vi "log analysis_gps.vi"() -> ()   [LabVIEW 2018] (continued)
0.0959,0.0768,0.1404,0.1455,4.9710,0f000001,0*c3454afa\n\tsystem status\tnormal 2 28.000000 0 0\trobot status\t312.499994\t49.181058\t10.952900\t-0.801069\t1.536454\t-28.115818\t0.278000\t0.033000\n\t\n15:25:42.1\tlog_raw\tgps_raw\t#INSPVAXA,USB3,0,48.5,FINESTEERING,2107,282360.150,02000000,471d,15824;INS_ALIGNMENT_COMPLETE,INS_RTKFIXED,37.37057265059,126.72436438219,10.9582,22.3000,-0.1754,0.2257,0.0186,-0.842848206,1.417409471,118.070069819,0.4412,0.2945,0.5472,0.1174,0.0950,0.0769,0.1402,0.1453,4.9710,0f000001,0*6a16ee00\n\tsystem status\tnormal 2 28.000000 0 0\trobot status\t312.617584\t49.099743\t10.958200\t-0.842848\t1.417409\t-28.070070\t0.252000\t0.062000\n\t\n15:25:42.6\tlog_raw\tgps_raw\t#INSPVAXA,USB3,0,48.5,FINESTEERING,2107,282360.650,02000000,471d,15824;INS_ALIGNMENT_COMPLETE,INS_RTKFIXED,37.37057191747,126.72436570845,10.9626,22.3000,-0.1784,0.2288,0.0199,-0.831650114,1.387719615,118.066694933,0.4412,0.2945,0.5472,0.1174,0.0950,0.0769,0.1402,0.1453,4.9710,0f000001,0*684747fc\n\tsystem status\tnormal 2 28.000000 0 0\trobot status\t312.735062\t49.018374\t10.962600\t-0.831650\t1.387720\t-28.066695\t0.284000\t0.026000\n\t\n15:25:43.1\tlog_raw\tgps_raw\t\tsystem status\tnormal 2 28.000000 0 0\trobot status\t312.853231\t48.935714\t10.967100\t-0.777129\t1.230060\t-28.133928\t0.295000\t-0.003000\n\t\n15:25:43.6\tlog_raw\tgps_raw\t#INSPVAXA,USB3,0,48.0,FINESTEERING,2107,282361.650,02000000,471d,15824;INS_ALIGNMENT_COMPLETE,INS_RTKFIXED,37.37057042530,126.72436839921,10.9712,22.3000,-0.1758,0.2244,0.0130,-0.782174586,1.064389692,118.205019127,0.4403,0.2942,0.5440,0.1166,0.0940,0.0770,0.1401,0.1452,4.9712,0f000001,0*a289776d\n\tsystem status\tnormal 2 28.000000 0 0\trobot status\t312.973405\t48.852757\t10.971200\t-0.782175\t1.064390\t-28.205019\t0.294000\t0.001000\n\t\n15:25:44.1\tlog_raw\tgps_raw\t#INSPVAXA,USB3,0,52.0,FINESTEERING,2107,282362.150,02000000,471d,15824;INS_ALIGNMENT_COMPLETE,INS_RTKFIXED,37.37056968661,126.72436971158,10.9754,22.3000,-0.1789,0.2227,0.0149,-0.712007512,1.145542222,118.217293959,0.4394,0.2937,0.5418,0.1158,0.0932,0.0771,0.1400,0.1450,4.9721,0f000001,0*3affd318\n\tsystem status\tnormal 2 28.000000 0 0\trobot status\t313.089653\t48.770770\t10.975400\t-0.712008\t1.145542\t-28.217294\t0.297000\t-0.006000\n\t\n15:25:44.6\tlog_raw\tgps_raw\t#INSPVAXA,USB3,0,52.0,FINESTEERING,2107,282362.650,02000000,471d,15824;INS_ALIGNMENT_COMPLETE,INS_RTKFIXED,37.37056893906,126.72437106065,10.9790,22.3000,-0.1744,0.2169,0.0071,-0.647011256,1.079419362,118.301292650,0.4394,0.2937,0.5418,0.1158,0.0932,0.0771,0.1400,0.1450,4.9721,0f000001,0*1e26d504\n\tsystem status\tnormal 2 28.000000 0 0\trobot status\t313.209151\t48.687799\t10.979000\t-0.647011\t1.079419\t-28.301293\t0.295000\t-0.013000\n\t\n15:25:45.1\tlog_raw\tgps_raw\t#INSPVAXA,USB3,0,52.5,FINESTEERING,2107,282363.150,02000000,471d,15824;INS_ALIGNMENT_COMPLETE,INS_RTKFIXED,37.37056818219,126.72437236922,10.9848,22.3000,-0.1880,0.2251,0.0164,-0.692024407,1.031121061,118.296623598,0.4394,0.2937,0.5418,0.1158,0.0932,0.0771,0.1400,0.1450,4.9721,0f000001,0*fbc0c197\n\tsystem status\tnormal 2 28.000000 0 0\trobot status\t313.325062\t48.603793\t10.984800\t-0.692024\t1.031121\t-28.296624\t0.300000\t0.002000\n\t\n15:25:45.6\tlog_raw\tgps_raw\t#INSPVAXA,USB3,0,52.5,FINESTEERING,2107,282363.650,02000000,471d,15824;INS_ALIGNMENT_COMPLETE,INS_RTKFIXED,37.37056736764,126.72437362581,10.9943,22.3000,-0.1838,0.2175,0.0187,-0.622586307,1.194821727,118.320117324,0.4394,0.2937,0.5418,0.1158,0.0932,0.0771,0.1400,0.1450,4.9721,0f000001,0*9ae06ad3\n\tsystem status\tnormal 2 28.000000 0 0\trobot status\t313.436369\t48.513387\t10.994300\t-0.622586\t1.194822\t-28.320117\t0.300000\t-0.003000\n\t\n15:25:46.1\tlog_raw\tgps_raw\t#INSPVAXA,USB3,0,46.5,FINESTEERING,2107,282364.150,02000000,471d,15824;INS_ALIGNMENT_COMPLETE,INS_RTKFIXED,37.37056657190,126.72437491440,11.0023,22.3000,-0.1853,0.2142,0.0193,-0.566287022,1.525613258,118.367713694,0.4907,0.3307,0.5859,0.1218,0.0978,0.0797,0.1410,0.1460,4.9751,0f000001,0*d0324f7d\n\tsystem status\tnormal 2 28.000000 0 0\trobot status\t313.550510\t48.425068\t11.002300\t-0.566287\t1.525613\t-28.367714\t0.297000\t-0.005000\n\t\n15:25:46.6\tlog_raw\tgps_raw\t#INSPVAXA,USB3,0,46.5,FINESTEERING,2107,282364.650,02000000,471d,15824;INS_ALIGNMENT_COMPLETE,INS_RTKFIXED,37.37056585214,126.72437630982,11.0047,22.3000,-0.1882,0.2248,0.0125,-0.569851294,1.528591804,118.479722218,0.4907,0.3307,0.5859,0.1218,0.0978,0.0797,0.1410,0.1460,4.9751,0f000001,0*9a426144\n\tsystem status\tnormal 2 28.000000 0 0\trobot status\t313.674114\t48.345181\t11.004700\t-0.569851\t1.528592\t-28.479722\t0.298000\t-0.001000\n\t\n15:25:47.1\tlog_raw\tgps_raw\t\tsystem status\tnormal 2 28.100000 0 0\trobot status\t313.794701\t48.266052\t11.006300\t-0.641358\t1.532620\t-28.563005\t0.302000\t-0.002000\n\t\n15:25:47.6\tlog_raw\tgps_raw\t#INSPVAXA,USB3,0,48.5,FINESTEERING,2107,282365.650,02000000,471d,15824;INS_ALIGNMENT_COMPLETE,INS_RTKFIXED,37.37056440793,126.72437904086,11.0071,22.3000,-0.1949,0.2319,0.0130,-0.541846536,1.457071221,118.616213426,0.4699,0.3127,0.5753,0.1175,0.0943,0.0785,0.1406,0.1454,4.9762,0f000001,0*40288813\n\tsystem status\tnormal 2 28.000000 0 0\trobot status\t313.916025\t48.184886\t11.007100\t-0.541847\t1.457071\t-28.616213\t0.302000\t-0.003000\n\t\n15:25:48.1\tlog_raw\tgps_raw\t\tsystem status\tnormal 2 28.000000 0 0\trobot status\t314.039024\t48.101275\t11.008300\t-0.456498\t1.022290\t-28.706558\t0.301000\t-0.003000\n\t\n15:25:48.6\tlog_raw\tgps_raw\t#INSPVAXA,USB3,0,51.0,FINESTEERING,2107,282366.650,02000000,471d,15824;INS_ALIGNMENT_COMPLETE,INS_RTKFIXED,37.37056291329,126.72438179261,11.0096,22.3000,-0.1917,0.2323,0.0080,-0.472728145,0.808367431,118.811459279,0.4569,0.3025,0.5669,0.1155,0.0932,0.0778,0.1406,0.1452,4.9769,0f000001,0*4a7ebce1\n\tsystem status\tnormal 2 28.000000 0 0\trobot status\t314.159770\t48.018995\t11.009600\t-0.472728\t0.808367\t-28.811459\t0.299000\t-0.008000\n\t\n15:25:49.1\tlog_raw\tgps_raw\t#INSPVAXA,USB3,0,52.5,FINESTEERING,2107,282367.150,02000000,471d,15824;INS_ALIGNMENT_COMPLETE,INS_RTKFIXED,37.37056215950,126.72438315251,11.0104,22.3000,-0.1905,0.2375,-0.0008,-0.383174802,0.623906770,118.905218595,0.4483,0.2967,0.5601,0.1147,0.0932,0.0773,0.1406,0.1452,4.9782,0f000001,0*ea495475\n\tsystem status\tnormal 2 28.000000 0 0\trobot status\t314.280228\t47.935332\t11.010400\t-0.383175\t0.623907\t-28.905219\t0.300000\t0.000000\n\t\n15:25:49.6\tlog_raw\tgps_raw\t#INSPVAXA,USB3,0,52.5,FINESTEERING,2107,282367.650,02000000,471d,15824;INS_ALIGNMENT_COMPLETE,INS_RTKFIXED,37.37056140665,126.72438451966,11.0108,22.3000,-0.1856,0.2294,0.0072,-0.390392792,0.506918836,119.017967456,0.4483,0.2967,0.5601,0.1147,0.0932,0.0773,0.1406,0.1452,4.9782,0f000001,0*a0cb1e22\n\tsystem status\tnormal 2 28.000000 0 0\trobot status\t314.401328\t47.851772\t11.010800\t-0.390393\t0.506919\t-29.017967\t0.295000\t-0.009000\n\t\n15:25:50.1\tlog_raw\tgps_raw\t#INSPVAXA,USB3,0,51.0,FINESTEERING,2107,282368.150,02000000,471d,15824;INS_ALIGNMENT_COMPLETE,INS_RTKFIXED,37.37056062590,126.72438588956,11.0109,22.3000,-0.1908,0.2384,0.0056,-0.245023334,0.482634279,119.176381690,0.4426,0.2937,0.5546,0.1146,0.0935,0.0770,0.1406,0.1452,4.9797,0f000001,0*61c8f471\n\tsystem status\tnormal 2 28.100000 0 0\trobot status\t314.522672\t47.765117\t11.010900\t-0.245023\t0.482634\t-29.176382\t0.301000\t-0.006000\n\t\n15:25:50.6\tlog_raw\tgps_raw\t\tsystem status\tnormal 2 28.000000 0 0\trobot status\t314.639459\t47.680741\t11.011100\t-0.155698\t0.523708\t-29.322196\t0.294000\t-0.012000\n\t\n15:25:51.1\tlog_raw\tgps_raw\t\tsystem status\tnormal 2 28.100000 0 0\trobot status\t314.757852\t47.595867\t11.011700\t-0.203616\t0.629165\t-29.462789\t0.298000\t-0.005000\n\t\n15:25:51.6\tlog_raw\tgps_raw\t\tsystem status\tnormal 2 28.000000 0 0\trobot status\t314.875057\t47.511316\t11.012200\t-0.096345\t0.825852\t-29.603097\t0.305000\t-0.002000\n\t\n15:25:52.1\tlog_raw\tgps_raw\t#INSPVAXA,USB3,0,49.0,FINESTEERING,2107,282370.150,02000000,471d,15824;INS_ALIGNMENT_COMPLETE,INS_RTKFIXED,37.37055758372,126.72439118773,11.0127,22.3000,-0.1993,0.2333,0.0205,-0.126523860,1.017645385,119.745065881,0.4369,0.2920,0.5469,0.1146,0.0935,0.0767,0.1404,0.1452,4.9818,0f000001,0*3c99dcc1\n\tsystem status\tnormal 2 28.100000 0 0\trobot status\t314.991975\t47.427464\t11.012700\t-0.126524\t1.017645\t-29.745066\t0.303000\t-0.007000\n\t\n15:25:52.6\tlog_raw\tgps_raw\t#INSPVAXA,USB3,0,49.0,FINESTEERING,2107,282370.650,02000000,471d,15824;INS_ALIGNMENT_COMPLETE,INS_RTKFIXED,37.37055683678,126.72439251585,11.0116,22.3000,-0.1882,0.2280,0.0157,-0.028794832,1.243937117,119.855600640,0.4369,0.2920,0.5469,0.1146,0.0935,0.0767,0.1404,0.1452,4.9818,0f000001,0*7496fdf6\n\tsystem status\tnormal 2 28.000000 0 0\trobot status\t315.109617\t47.344561\t11.011600\t-0.028795\t1.243937\t-29.855601\t0.298000\t-0.003000\n\t\n15:25:53.1\tlog_raw\tgps_raw\t#INSPVAXA,USB3,0,50.0,FINESTEERING,2107,282371.150,02000000,471d,15824;INS_ALIGNMENT_COMPLETE,INS_RTKFIXED,37.37055608815,126.72439385420,11.0119,22.3000,-0.1947,0.2327,0.0119,-0.172585460,1.434683423,119.971021632,0.4362,0.2920,0.5445,0.1145,0.0933,0.0767,0.1403,0.1451,4.9828,0f000001,0*21210484\n\tsystem status\tnormal 2 28.000000 0 0\trobot status\t315.228166\t47.261470\t11.011900\t-0.172585\t1.434683\t-29.971022\t0.298000\t-0.006000\n\t\n15:25:53.6\tlog_raw\tgps_raw\t\tsystem status\tnormal 2 28.000000 0 0\trobot status\t315.345773\t47.177357\t11.014400\t-0.196990\t1.571426\t-30.064709\t0.300000\t-0.003000\n\t\n15:25:54.1\tlog_raw\tgps_raw\t#INSPVAXA,USB3,0,51.5,FINESTEERING,2107,282372.150,02000000,471d,15824;INS_ALIGNMENT_COMPLETE,INS_RTKFIXED,37.37055456936,126.72439651011,11.0164,22.3000,-0.1955,0.2409,0.0111,-0.219662540,1.523066088,120.209141844,0.4362,0.2922,0.5426,0.1144,0.0930,0.0767,0.1402,0.1451,4.9843,0f000001,0*f3fda870\n\tsystem status\tnormal 2 28.000000 0 0\trobot status\t315.463422\t47.092898\t11.016400\t-0.219663\t1.523066\t-30.209142\t0.300000\t-0.003000\n\t\n15:25:54.6\tlog_raw\tgps_raw\t#INSPVAXA,USB3,0,51.5,FINESTEERING,2107,282372.650,02000000,471d,15824;INS_ALIGNMENT_COMPLETE,INS_RTKFIXED,37.37055382453,126.72439783430,11.0178,22.3000,-0.1964,0.2384,0.0010,-0.282113578,1.525554977,120.284642738,0.4362,0.2922,0.5426,0.1144,0.0930,0.0767,0.1402,0.1451,4.9843,0f000001,0*1248182f\n\tsystem status\tnormal 2 28.000000 0 0\trobot status\t315.580717\t47.010229\t11.017800\t-0.282114\t1.525555\t-30.284643\t0.304000\t-0.003000\n\t\n15:25:55.1\tlog_raw\tgps_raw\t\tsystem status\tnormal 2 28.000000 0 0\trobot status\t315.696671\t46.927649\t11.019900\t-0.369047\t1.556384\t-30.408820\t0.302000\t-0.002000\n\t\n15:25:55.6\tlog_raw\tgps_raw\t\tsystem status\tnormal 2 28.000000 0 0\trobot status\t315.812317\t46.846568\t11.022200\t-0.486619\t1.626980\t-30.509329\t0.299000\t-0.001000\n\t\n15:25:56.1\tlog_raw\tgps_raw\t#INSPVAXA,USB3,0,48.5,FINESTEERING,2107,282374.150,02000000,471d,15824;INS_ALIGNMENT_COMPLETE,INS_RTKFIXED,37.37055158865,126.72440177016,11.0240,22.3000,-0.1992,0.2398,-0.0010,-0.425522010,1.592578563,120.559312340,0.4364,0.2923,0.5406,0.1141,0.0924,0.0768,0.1401,0.1450,4.9874,0f000001,0*101c3bdb\n\tsystem status\tnormal 2 28.000000 0 0\trobot status\t315.929349\t46.762068\t11.024000\t-0.425522\t1.592579\t-30.559312\t0.299000\t0.000000\n\t\n15:25:56.6\tlog_raw\tgps_raw\t\tsystem status\tnormal 2 28.000000 0 0\trobot status\t316.042991\t46.678607\t11.025500\t-0.387054\t1.725149\t-30.587652\t0.302000\t0.005000\n\t\n15:25:57.1\tlog_raw\tgps_raw\t#INSPVAXA,USB3,0,51.0,FINESTEERING,2107,282375.150,02000000,471d,15824;INS_ALIGNMENT_COMPLETE,INS_RTKFIXED,37.37055007830,126.72440434973,11.0274,22.3000,-0.1945,0.2378,0.0125,-0.376290277,1.647280363,120.637326967,0.4364,0.2922,0.5400,0.1139,0.0922,0.0768,0.1401,0.1450,4.9889,0f000001,0*67dcfdd6\n\tsystem status\tnormal 2 28.000000 0 0\trobot status\t316.157843\t46.594434\t11.027400\t-0.376290\t1.647280\t-30.637327\t0.300000\t0.005000\n\t\n15:25:57.6\tlog_raw\tgps_raw\t\tsystem status\tnormal 2 28.000000 0 0\trobot status\t316.274584\t46.510665\t11.030000\t-0.408630\t1.445980\t-30.686561\t0.300000\t0.000000\n\t\n15:25:58.1\tlog_raw\tgps_raw\t#INSPVAXA,USB3,0,50.5,FINESTEERING,2107,282376.150,02000000,471d,15824;INS_ALIGNMENT_COMPLETE,INS_RTKFIXED,37.37054852803,126.72440700509,11.0323,22.3000,-0.1988,0.2410,0.0047,-0.545420611,1.322594282,120.751487308,0.4364,0.2922,0.5400,0.1139,0.0922,0.0768,0.1401,0.1450,4.9889,0f000001,0*a32cf91e\n\tsystem status\tnormal 2 28.100000 0 0\trobot status\t316.393051\t46.422369\t11.032300\t-0.545421\t1.322594\t-30.751487\t0.300000\t-0.002000\n\t\n15:25:58.6\tlog_raw\tgps_raw\t\tsystem status\tnormal 2 28.100000 0 0\trobot status\t316.511188\t46.324929\t11.035600\t-0.547076\t1.168807\t-30.825969\t0.296000\t-0.001000\n\t\n15:25:59.1\tlog_raw\tgps_raw\t#INSPVAXA,USB3,0,56.0,FINESTEERING,2107,282377.150,02000000,471d,15824;INS_ALIGNMENT_COMPLETE,INS_RTKFIXED,37.37054676587,126.72440967582,11.0390,22.3000,-0.1999,0.2394,0.0134,-0.643659159,1.057296684,120.890681987,0.4364,0.2922,0.5400,0.1139,0.0922,0.0768,0.1401,0.1450,4.9889,0f000001,0*19d68dee\n\tsystem status\tnormal 2 28.000000 0 0\trobot status\t316.629619\t46.226787\t11.039000\t-0.643659\t1.057297\t-30.890682\t0.302000\t-0.001000\n\t\n15:25:59.6\tlog_raw\tgps_raw\t\tsystem status\tnormal 2 28.000000 0 0\trobot status\t316.748960\t46.127007\t11.042800\t-0.703333\t0.970865\t-30.940874\t0.301000\t-0.001000\n\t\n15:26:00.1\tlog_raw\tgps_raw\t\tsystem status\tnormal 2 28.000000 0 0\trobot status\t316.865490\t46.034320\t11.046500\t-0.687765\t1.023030\t-30.956072\t0.298000\t0.006000\n\t\n15:26:00.6\tlog_raw\tgps_raw\t\tsystem status\tnormal 2 28.000000 0 0\trobot status\t316.977105\t45.965920\t11.049700\t-0.782262\t1.108092\t-31.008444\t0.298000\t0.007000\n\t\n15:26:01.1\tlog_raw\tgps_raw\t\tsystem status\tnormal 2 28.000000 0 0\trobot status\t317.090034\t45.892807\t11.051400\t-0.771591\t1.089832\t-31.020335\t0.298000\t0.004000\n\t\n15:26:01.6\tlog_raw\tgps_raw\t\tsystem status\tnormal 2 28.000000 0 0\trobot status\t317.206952\t45.812611\t11.052200\t-0.744284\t1.080656\t-31.021960\t0.298000\t0.005000\n\t\n15:26:02.1\tlog_raw\tgps_raw\t#INSPVAXA,USB3,0,51.5,FINESTEERING,2107,282380.150,02000000,471d,15824;INS_ALIGNMENT_COMPLETE,INS_RTKFIXED,37.37054231634,126.72441746453,11.0545,22.3000,-0.1950,0.2290,0.0101,-0.779433924,1.099591646,120.976695611,0.4675,0.3093,0.5930,0.1184,0.0970,0.0772,0.1414,0.1460,4.9947,0f000001,0*af9d06d5\n\tsystem status\tnormal 2 28.000000 0 0\trobot status\t317.319531\t45.732932\t11.054500\t-0.779434\t1.099592\t-30.976696\t0.347000\t-0.076000\n\t\n15:26:02.6\tlog_raw\tgps_raw\t\tsystem status\tnormal 2 28.000000 0 0\trobot status\t317.432586\t45.649792\t11.057900\t-0.839077\t1.246140\t-30.921525\t0.333000\t-0.061000\n\t\n15:26:03.1\tlog_raw\tgps_raw\t\tsystem status\tnormal 2 28.000000 0 0\trobot status\t317.550663\t45.559859\t11.060900\t-0.816495\t1.347080\t-30.908043\t0.247000\t0.059000\n\t\n15:26:03.6\tlog_raw\tgps_raw\t\tsystem status\tnormal 2 28.000000 0 0\trobot status\t317.667916\t45.463494\t11.064400\t-0.887391\t1.440630\t-30.847180\t0.259000\t0.059000\n\t\n15:26:04.1\tlog_raw\tgps_raw\t\tsystem status\tnormal 2 28.000000 0 0\trobot status\t317.784177\t45.372249\t11.068000\t-0.895954\t1.399755\t-30.787069\t0.348000\t-0.082000\n\t\n15:26:04.6\tlog_raw\tgps_raw\t\tsystem status\tnormal 2 28.000000 0 0\trobot status\t317.897989\t45.297471\t11.072100\t-0.868246\t1.325384\t-30.710013\t0.268000\t0.039000\n\t\n15:26:05.1\tlog_raw\tgps_raw\t\tsystem status\tnormal 2 28.000000 0 0\trobot status\t318.012551\t45.219365\t11.077100\t-0.737707\t1.224592\t-30.609820\t0.274000\t0.027000\n\t\n15:26:05.6\tlog_raw\tgps_raw\t\tsystem status\tnormal 2 28.000000 0 0\trobot status\t318.126528\t45.138525\t11.083300\t-0.713978\t1.140149\t-30.534342\t0.347000\t-0.089000\n\t\n15:26:06.1\tlog_raw\tgps_raw\t\tsystem status\tnormal 2 28.000000 0 0\trobot status\t318.241724\t45.053708\t11.088800\t-0.781618\t1.201474\t-30.564329\t0.257000\t0.043000\n\t\n15:26:06.6\tlog_raw\tgps_raw\t\tsystem status\tnormal 2 28.000000 0 0\trobot status\t318.360025\t44.958001\t11.094400\t-0.854089\t1.233668\t-30.586480\t0.294000\t-0.009000\n\t\n15:26:07.1\tlog_raw\tgps_raw\t\tsystem status\tnormal 2 28.000000 0 0\trobot status\t318.473921\t44.868063\t11.099900\t-0.830682\t1.383003\t-30.588756\t0.296000\t-0.005000\n\t\n15:26:07.6\tlog_raw\tgps_raw\t\tsystem status\tnormal 2 28.000000 0 0\trobot status\t318.583583\t44.793348\t11.105400\t-0.688458\t1.421619\t-30.626819\t0.293000\t-0.015000\n\t\n15:26:08.1\tlog_raw\tgps_raw\t\tsystem status\tnormal 2 28.100000 0 0\trobot status\t318.695376\t44.715083\t11.110500\t-0.621575\t1.442793\t-30.687734\t0.298000\t-0.012000\n\t\n15:26:08.6\tlog_raw\tgps_raw\t\tsystem status\tnormal 2 28.000000 0 0\trobot status\t318.807113\t44.634368\t11.117200\t-0.699288\t1.578888\t-30.729025\t0.291000\t-0.015000\n\t\n15:26:09.1\tlog_raw\tgps_raw\t\tsystem status\tnormal 2 28.000000 0 0\trobot status\t318.919028\t44.547774\t11.125000\t-0.655876\t1.582589\t-30.761990\t0.296000\t-0.011000\n\t\n15:26:09.6\tlog_raw\tgps_raw\t\tsystem status\tnormal 2 28.000000 0 0\trobot status\t319.034952\t44.448217\t11.133200\t-0.642971\t1.523191\t-30.813225\t0.297000\t-0.014000\n\t\n15:26:10.1\tlog_raw\tgps_raw\t\tsystem status\tnormal 2 28.100000 0 0\trobot status\t319.150075\t44.353379\t11.141000\t-0.602027\t1.630659\t-30.864026\t0.299000\t-0.010000\n\t\n15:26:10.6\tlog_raw\tgps_raw\t\tsystem status\tnormal 2 28.000000 0 0\trobot status\t319.261183\t44.276146\t11.147400\t-0.528294\t1.572516\t-30.922958\t0.298000\t0.000000\n\t\n15:26:11.1\tlog_raw\tgps_raw\t\tsystem status\tnormal 2 28.000000 0 0\trobot status\t319.374097\t44.194709\t11.154200\t-0.383438\t1.395307\t-31.049945\t0.299000\t0.000000\n\t\n15:26:11.7\tlog_raw\tgps_raw\t\tsystem status\tnormal 2 28.000000 0 0\trobot status\t319.488062\t44.108823\t11.159600\t-0.206184\t1.242922\t-31.135620\t0.292000\t-0.007000\n\t\n15:26:12.1\tlog_raw\tgps_raw\t\tsystem status\tnormal 2 28.000000 0 0\trobot status\t319.601847\t44.022896\t11.165400\t-0.173678\t1.198516\t-31.218283\t0.294000\t-0.003000\n\t\n15:26:12.7\tlog_raw\tgps_raw\t\tsystem status\tnormal 2 28.000000 0 0\trobot status\t319.716831\t43.937029\t11.170500\t-0.251651\t1.246692\t-31.292043\t0.296000\t-0.005000\n\t\n15:26:13.2\tlog_raw\tgps_raw\t\tsystem status\tnormal 2 28.000000 0 0\trobot status\t319.831302\t43.849544\t11.176100\t-0.193272\t1.314153\t-31.350185\t0.297000\t-0.010000\n\t\n15:26:13.7\tlog_raw\tgps_raw\t\tsystem status\tnormal 2 28.100000 0 0\trobot status\t319.948465\t43.760462\t11.184100\t-0.050481\t1.406412\t-31.381709\t0.296000\t-0.006000\n\t\n15:26:14.2\tlog_raw\tgps_raw\t\tsystem status\tnormal 2 28.000000 0 0\trobot status\t320.061943\t43.672961\t11.191600\t-0.042890\t1.719894\t-31.413597\t0.301000\t0.003000\n\t\n15:26:14.7\tlog_raw\tgps_raw\t\tsystem status\tnormal 2 28.000000 0 0\trobot status\t320.175399\t43.584307\t11.196800\t-0.016793\t1.699514\t-31.492516\t0.297000\t0.001000\n\t\n15:26:15.2\tlog_raw\tgps_raw\t\tsystem status\tnormal 2 28.000000 0 0\trobot status\t320.290219\t43.495259\t11.202000\t-0.158228\t1.837171\t-31.577321\t0.304000\t0.002000\n\t\n15:26:15.7\tlog_raw\tgps_raw\t\tsystem status\tnormal 2 28.000000 0 0\trobot status\t320.403890\t43.407183\t11.206700\t-0.121054\t1.987495\t-31.576185\t0.295000\t0.005000\n\t\n15:26:16.2\tlog_raw\tgps_raw\t\tsystem status\tnormal 2 28.000000 0 0\trobot status\t320.518730\t43.318566\t11.212000\t-0.192713\t1.993255\t-31.623743\t0.300000\t0.008000\n\t\n15:26:16.7\tlog_raw\tgps_raw\t\tsystem status\tnormal 2 28.000000 0 0\trobot status\t320.635793\t43.229652\t11.218000\t-0.297416\t1.926594\t-31.642658\t0.300000\t-0.001000\n\t\n15:26:17.2\tlog_raw\tgps_raw\t\tsystem status\tnormal 2 28.000000 0 0\trobot status\t320.751780\t43.139819\t11.224000\t-0.293698\t2.010038\t-31.639513\t0.303000\t0.005000\n\t\n15:26:17.7\tlog_raw\tgps_raw\t\tsystem status\tnormal 2 28.000000 0 0\trobot status\t320.866959\t43.051021\t11.228800\t-0.252225\t1.853648\t-31.644727\t0.312000\t0.000000\n\t\n15:26:18.2\tlog_raw\tgps_raw\t#INSPVAXA,USB3,0,53.0,FINESTEERING,2107,282396.200,02000000,471d,15824;INS_ALIGNMENT_COMPLETE,INS_RTKFIXED,37.37051727534,126.72445893614,11.2346,22.3000,-0.2149,0.2448,0.0105,-0.230381953,1.670919034,121.706042723,0.4454,0.2945,0.5444,0.1167,0.0933,0.0771,0.1396,0.1448,5.0169,0f000001,0*e3a105a8\n\tsystem status\tnormal 2 28.000000 0 0\trobot status\t320.993018\t42.953626\t11.234600\t-0.230382\t1.670919\t-31.706043\t0.300000\t0.002000\n\t\n15:26:18.7\tlog_raw\tgps_raw\t\tsystem status\tnormal 2 28.000000 0 0\trobot status\t321.098911\t42.873834\t11.238800\t-0.374769\t1.739257\t-31.716837\t0.308000\t0.000000\n\t\n15:26:19.2\tlog_raw\tgps_raw\t\tsystem status\tnormal 2 28.000000 0 0\trobot status\t321.215034\t42.784862\t11.243700\t-0.317896\t1.583496\t-31.672183\t0.300000\t0.004000\n\t\n15:26:19.7\tlog_raw\tgps_raw\t\tsystem status\tnormal 2 28.000000 0 0\trobot status\t321.328995\t42.697954\t11.248100\t-0.292274\t1.413082\t-31.609032\t0.276000\t0.045000\n\t\n15:26:20.2\tlog_raw\tgps_raw\t\tsystem status\tnormal 2 28.000000 0 0\trobot status\t321.443612\t42.609385\t11.252400\t-0.217796\t1.413222\t-31.467886\t0.278000\t0.035000\n\t\n15:26:20.7\tlog_raw\tgps_raw\t\tsystem status\tnormal 2 28.000000 0 0\trobot status\t321.559858\t42.520982\t11.255400\t-0.213988\t1.321824\t-31.289097\t0.239000\t0.085000\n\t\n15:26:21.2\tlog_raw\tgps_raw\t\tsystem status\tnormal 2 28.000000 0 0\trobot status\t321.673832\t42.434194\t11.258900\t-0.220342\t1.308636\t-31.041861\t0.293000\t0.016000\n\t\n15:26:21.7\tlog_raw\tgps_raw\t#INSPVAXA,USB3,0,52.5,FINESTEERING,2107,282399.700,02000000,471d,15824;INS_ALIGNMENT_COMPLETE,INS_RTKFIXED,37.37051173912,126.72446803450,11.2629,22.3000,-0.2157,0.2432,0.0104,-0.126649868,1.183808073,120.810959551,0.4494,0.2941,0.5444,0.1155,0.0921,0.0775,0.1396,0.1447,5.0208,0f000001,0*57a15611\n\tsystem status\tnormal 2 28.000000 0 0\trobot status\t321.798936\t42.339160\t11.262900\t-0.126650\t1.183808\t-30.810960\t0.289000\t0.028000\n\t\n15:26:22.2\tlog_raw\tgps_raw\t#INSPVAXA,USB3,0,51.5,FINESTEERING,2107,282400.200,02000000,471d,15824;INS_ALIGNMENT_COMPLETE,INS_RTKFIXED,37.37051098079,126.72446931042,11.2663,22.3000,-0.2068,0.2423,0.0047,-0.194058602,1.122857123,120.589823258,0.4487,0.2937,0.5447,0.1150,0.0920,0.0775,0.1397,0.1447,5.0216,0f000001,0*c9fba93a\n\tsystem status\tnormal 2 28.000000 0 0\trobot status\t321.911955\t42.254993\t11.266300\t-0.194059\t1.122857\t-30.589823\t0.284000\t0.024000\n\t\n15:26:22.7\tlog_raw\tgps_raw\t#INSPVAXA,USB3,0,51.5,FINESTEERING,2107,282400.700,02000000,471d,15824;INS_ALIGNMENT_COMPLETE,INS_RTKFIXED,37.37051023771,126.72447057615,11.2691,22.3000,-0.2018,0.2421,0.0003,-0.178083607,1.252069735,120.254195677,0.4487,0.2937,0.5447,0.1150,0.0920,0.0775,0.1397,0.1447,5.0216,0f000001,0*c019cdcb\n\tsystem status\tnormal 2 28.000000 0 0\trobot status\t322.024071\t42.172518\t11.269100\t-0.178084\t1.252070\t-30.254196\t0.274000\t0.045000\n\t\n15:26:23.2\tlog_raw\tgps_raw\t\tsystem status\tnormal 2 27.900000 0 0\trobot status\t322.123807\t42.099686\t11.272300\t-0.161582\t1.307019\t-29.978398\t0.308000\t-0.002000\n\t\n15:26:23.7\tlog_raw\tgps_raw\t\tsystem status\tnormal 2 28.000000 0 0\trobot status\t322.238275\t42.017640\t11.276500\t-0.061771\t1.314666\t-29.738310\t0.279000\t0.036000\n\t\n15:26:24.2\tlog_raw\tgps_raw\t\tsystem status\tnormal 2 28.000000 0 0\trobot status\t322.352343\t41.937206\t11.280200\t-0.171851\t1.578799\t-29.480802\t0.412000\t-0.174000\n\t\n15:26:24.7\tlog_raw\tgps_raw\t#INSPVAXA,USB3,0,52.0,FINESTEERING,2107,282402.700,02000000,471d,15824;INS_ALIGNMENT_COMPLETE,INS_RTKFIXED,37.37050732665,126.72447567900,11.2840,22.3000,-0.1846,0.2304,0.0147,-0.197464539,1.720744587,119.244672502,0.4474,0.2933,0.5456,0.1143,0.0919,0.0775,0.1398,0.1447,5.0227,0f000001,0*ef6b078e\n\tsystem status\tnormal 2 28.000000 0 0\trobot status\t322.476073\t41.849418\t11.284000\t-0.197465\t1.720745\t-29.244673\t0.290000\t0.025000\n\t\n15:26:25.2\tlog_raw\tgps_raw\t\tsystem status\tnormal 2 28.000000 0 0\trobot status\t322.579374\t41.776811\t11.285800\t-0.232380\t1.437411\t-29.131770\t0.279000\t0.023000\n\t\n15:26:25.7\tlog_raw\tgps_raw\t#INSPVAXA,USB3,0,51.0,FINESTEERING,2107,282403.700,02000000,471d,15824;INS_ALIGNMENT_COMPLETE,INS_RTKFIXED,37.37050587454,126.72447826035,11.2883,22.3000,-0.1895,0.2228,0.0117,-0.041463128,1.413686081,119.013719695,0.4466,0.2931,0.5458,0.1142,0.0920,0.0774,0.1398,0.1448,5.0238,0f000001,0*aa5be0c8\n\tsystem status\tnormal 2 28.000000 0 0\trobot status\t322.704725\t41.688247\t11.288300\t-0.041463\t1.413686\t-29.013720\t0.280000\t0.023000\n\t\n15:26:26.2\tlog_raw\tgps_raw\t\tsystem status\tnormal 2 28.000000 0 0\trobot status\t322.807611\t41.615847\t11.290100\t0.014448\t1.226451\t-28.973744\t0.269000\t0.043000\n\t\n15:26:26.7\tlog_raw\tgps_raw\t\tsystem status\tnormal 2 28.000000 0 0\trobot status\t322.922819\t41.536064\t11.293200\t-0.047041\t1.026542\t-28.942700\t0.261000\t0.062000\n\t\n15:26:27.2\tlog_raw\tgps_raw\t#INSPVAXA,USB3,0,53.0,FINESTEERING,2107,282405.200,02000000,471d,15824;INS_ALIGNMENT_COMPLETE,INS_RTKFIXED,37.37050369833,126.72448216938,11.2960,22.3000,-0.1948,0.2280,0.0025,-0.062260759,1.020577864,118.930310663,0.4445,0.2927,0.5458,0.1142,0.0920,0.0773,0.1398,0.1448,5.0258,0f000001,0*8918fe41\n\tsystem status\tnormal 2 28.000000 0 0\trobot status\t323.050980\t41.446708\t11.296000\t-0.062261\t1.020578\t-28.930311\t0.346000\t-0.071000\n\t\n15:26:27.7\tlog_raw\tgps_raw\t\tsystem status\tnormal 2 28.000000 0 0\trobot status\t323.157063\t41.374190\t11.297300\t8.474600E-5\t0.954576\t-28.962463\t0.297000\t-0.005000\n\t\n15:26:28.2\tlog_raw\tgps_raw\t#INSPVAXA,USB3,0,49.0,FINESTEERING,2107,282406.200,02000000,471d,15824;INS_ALIGNMENT_COMPLETE,INS_RTKFIXED,37.37050223457,126.72448478438,11.2989,22.3000,-0.1940,0.2271,0.0004,0.403911528,1.100287176,119.003406163,0.4431,0.2925,0.5454,0.1141,0.0922,0.0772,0.1398,0.1448,5.0266,0f000001,0*9acaefa2\n\tsystem status\tnormal 2 28.100000 0 0\trobot status\t323.282613\t41.284244\t11.298900\t0.403912\t1.100287\t-29.003406\t0.308000\t-0.008000\n\t\n15:26:28.7\tlog_raw\tgps_raw\t#INSPVAXA,USB3,0,49.0,FINESTEERING,2107,282406.700,02000000,471d,15824;INS_ALIGNMENT_COMPLETE,INS_RTKFIXED,37.37050154645,126.72448605087,11.3007,22.3000,-0.1906,0.2211,-0.0024,0.198399759,1.155504209,119.019429949,0.4431,0.2925,0.5454,0.1141,0.0922,0.0772,0.1398,0.1448,5.0266,0f000001,0*2b05d55f\n\tsystem status\tnormal 2 28.000000 0 0\trobot status\t323.394796\t41.207869\t11.300700\t0.198400\t1.155504\t-29.019430\t0.300000\t-0.005000\n\t\n15:26:29.2\tlog_raw\tgps_raw\t#INSPVAXA,USB3,0,49.5,FINESTEERING,2107,282407.200,02000000,471d,15824;INS_ALIGNMENT_COMPLETE,INS_RTKFIXED,37.37050082511,126.72448737364,11.3024,22.3000,-0.1843,0.2252,0.0031,0.001432132,1.154226626,118.999213590,0.4420,0.2924,0.5450,0.1140,0.0921,0.0771,0.1398,0.1448,5.0273,0f000001,0*acf3bb7b\n\tsystem status\tnormal 2 28.100000 0 0\trobot status\t323.511965\t41.127807\t11.302400\t0.001432\t1.154227\t-28.999214\t0.299000\t-0.008000\n\t\n15:26:29.7\tlog_raw\tgps_raw\t#INSPVAXA,USB3,0,49.5,FINESTEERING,2107,282407.700,02000000,471d,15824;INS_ALIGNMENT_COMPLETE,INS_RTKFIXED,37.37050009749,126.72448866196,11.3047,22.3000,-0.1922,0.2264,0.0013,0.031954534,1.373571777,119.029897417,0.4420,0.2924,0.5450,0.1140,0.0921,0.0771,0.1398,0.1448,5.0273,0f000001,0*4feaee25\n\tsystem status\tnormal 2 28.000000 0 0\trobot status\t323.626082\t41.047048\t11.304700\t0.031955\t1.373572\t-29.029897\t0.304000\t-0.002000\n\t\n15:26:30.2\tlog_raw\tgps_raw\t\tsystem status\tnormal 2 28.000000 0 0\trobot status\t323.727747\t40.974413\t11.307100\t0.072493\t1.528107\t-29.075426\t0.301000\t-0.002000\n\t\n15:26:30.7\tlog_raw\tgps_raw\t#INSPVAXA,USB3,0,49.5,FINESTEERING,2107,282408.700,02000000,471d,15824;INS_ALIGNMENT_COMPLETE,INS_RTKFIXED,37.37049862952,126.72449128459,11.3098,22.3000,-0.1866,0.2253,0.0102,0.047127376,1.614716400,119.167288999,0.4410,0.2922,0.5445,0.1140,0.0921,0.0770,0.1398,0.1448,5.0281,0f000001,0*196c2f22\n\tsystem status\tnormal 2 28.000000 0 0\trobot status\t323.858391\t40.884117\t11.309800\t0.047127\t1.614716\t-29.167289\t0.303000\t-0.012000\n\t\n15:26:31.2\tlog_raw\tgps_raw\t#INSPVAXA,USB3,0,47.5,FINESTEERING,2107,282409.200,02000000,471d,15824;INS_ALIGNMENT_COMPLETE,INS_RTKFIXED,37.37049789341,126.72449262767,11.3125,22.3000,-0.1999,0.2359,0.0079,-0.178457330,1.548416838,119.244672995,0.4408,0.2923,0.5442,0.1140,0.0922,0.0770,0.1398,0.1448,5.0295,0f000001,0*fefe7bbe\n\tsystem status\tnormal 2 28.000000 0 0\trobot status\t323.977358\t40.802415\t11.312500\t-0.178457\t1.548417\t-29.244673\t0.302000\t0.000000\n\t\n15:26:31.7\tlog_raw\tgps_raw\t\tsystem status\tnormal 2 28.100000 0 0\trobot status\t324.083822\t40.729055\t11.315700\t-0.361621\t1.540910\t-29.327056\t0.299000\t-0.004000\n\t\n15:26:32.2\tlog_raw\tgps_raw\t\tsystem status\tnormal 2 28.000000 0 0\trobot status\t324.201244\t40.646211\t11.320200\t-0.395668\t1.402025\t-29.391054\t0.295000\t-0.006000\n\t\n15:26:32.7\tlog_raw\tgps_raw\t#INSPVAXA,USB3,0,49.0,FINESTEERING,2107,282410.700,02000000,471d,15824;INS_ALIGNMENT_COMPLETE,INS_RTKFIXED,37.37049566854,126.72449665280,11.3239,22.3000,-0.1868,0.2363,0.0016,-0.505574846,1.345277164,119.533703259,0.4402,0.2922,0.5436,0.1139,0.0922,0.0769,0.1398,0.1447,5.0311,0f000001,0*6012c6b0\n\tsystem status\tnormal 2 28.000000 0 0\trobot status\t324.333898\t40.555475\t11.323900\t-0.505575\t1.345277\t-29.533703\t0.305000\t-0.006000\n\t\n15:26:33.2\tlog_raw\tgps_raw\t#INSPVAXA,USB3,0,50.0,FINESTEERING,2107,282411.200,02000000,471d,15824;INS_ALIGNMENT_COMPLETE,INS_RTKFIXED,37.37049487353,126.72449799751,11.3279,22.3000,-0.1792,0.2394,0.0156,-0.401695145,1.333527826,119.633898753,0.4402,0.2922,0.5436,0.1139,0.0922,0.0769,0.1398,0.1447,5.0311,0f000001,0*2fc42002\n\tsystem status\tnormal 2 28.000000 0 0\trobot status\t324.453010\t40.467237\t11.327900\t-0.401695\t1.333528\t-29.633899\t0.302000\t-0.006000\n\t\n15:26:33.7\tlog_raw\tgps_raw\t#INSPVAXA,USB3,0,50.0,FINESTEERING,2107,282411.700,02000000,471d,15824;INS_ALIGNMENT_COMPLETE,INS_RTKFIXED,37.37049401462,126.72449935015,11.3332,22.3000,-0.1865,0.2337,0.0135,-0.484899234,1.283665048,119.740703059,0.4402,0.2922,0.5436,0.1139,0.0922,0.0769,0.1398,0.1447,5.0311,0f000001,0*1d33eb73\n\tsystem status\tnormal 2 28.000000 0 0\trobot status\t324.572825\t40.371906\t11.333200\t-0.484899\t1.283665\t-29.740703\t0.299000\t-0.008000\n\t\n15:26:34.2\tlog_raw\tgps_raw\t#INSPVAXA,USB3,0,45.5,FINESTEERING,2107,282412.200,02000000,471d,15824;INS_ALIGNMENT_COMPLETE,INS_RTKFIXED,37.37049319930,126.72450071545,11.3390,22.3000,-0.1883,0.2399,0.0132,-0.511269715,1.109019547,119.856142336,0.4907,0.3298,0.5890,0.1210,0.0979,0.0793,0.1408,0.1457,5.0340,0f000001,0*b0282710\n\tsystem status\tnormal 2 28.000000 0 0\trobot status\t324.693761\t40.281414\t11.339000\t-0.511270\t1.109020\t-29.856142\t0.303000\t-0.008000\n\t\n15:26:34.7\tlog_raw\tgps_raw\t#INSPVAXA,USB3,0,45.5,FINESTEERING,2107,282412.700,02000000,471d,15824;INS_ALIGNMENT_COMPLETE,INS_RTKFIXED,37.37049251112,126.72450203682,11.3445,22.3000,-0.1885,0.2438,0.0204,-0.533735812,1.097181007,119.915108239,0.4907,0.3298,0.5890,0.1210,0.0979,0.0793,0.1408,0.1457,5.0340,0f000001,0*9a141504\n\tsystem status\tnormal 2 28.000000 0 0\trobot status\t324.810806\t40.205032\t11.344500\t-0.533736\t1.097181\t-29.915108\t0.304000\t-0.001000\n\t\n15:26:35.2\tlog_raw\tgps_raw\t#INSPVAXA,USB3,0,46.5,FINESTEERING,2107,282413.200,02000000,471d,15824;INS_ALIGNMENT_COMPLETE,INS_RTKFIXED,37.37049180169,126.72450336418,11.3490,22.3000,-0.1814,0.2477,0.0198,-0.567250496,1.161668497,119.990441604,0.4687,0.3125,0.5782,0.1173,0.0947,0.0780,0.1403,0.1452,5.0347,0f000001,0*907c6878\n\tsystem status\tnormal 2 28.000000 0 0\trobot status\t324.928381\t40.126291\t11.349000\t-0.567250\t1.161668\t-29.990442\t0.304000\t0.007000\n\t\n15:26:35.7\tlog_raw\tgps_raw\t#INSPVAXA,USB3,0,46.5,FINESTEERING,2107,282413.700,02000000,471d,15824;INS_ALIGNMENT_COMPLETE,INS_RTKFIXED,37.37049106798,126.72450467966,11.3532,22.3000,-0.1907,0.2386,0.0196,-0.535844359,1.216959402,120.030591907,0.4687,0.3125,0.5782,0.1173,0.0947,0.0780,0.1403,0.1452,5.0347,0f000001,0*639bb67e\n\tsystem status\tnormal 2 28.000000 0 0\trobot status\t325.044904\t40.044856\t11.353200\t-0.535844\t1.216959\t-30.030592\t0.300000\t0.004000\n\t\n15:26:36.2\tlog_raw\tgps_raw\t#INSPVAXA,USB3,0,51.5,FINESTEERING,2107,282414.200,02000000,471d,15824;INS_ALIGNMENT_COMPLETE,INS_RTKFIXED,37.37049032617,126.72450602273,11.3581,22.3000,-0.1924,0.2499,0.0107,-0.616512696,1.220090147,120.041431319,0.4551,0.3027,0.5696,0.1158,0.0939,0.0773,0.1402,0.1450,5.0349,0f000001,0*41bc56e6\n\tsystem status\tnormal 2 28.000000 0 0\trobot status\t325.163871\t39.962522\t11.358100\t-0.616513\t1.220090\t-30.041431\t0.298000\t0.003000\n\t\n15:26:36.7\tlog_raw\tgps_raw\t#INSPVAXA,USB3,0,51.5,FINESTEERING,2107,282414.700,02000000,471d,15824;INS_ALIGNMENT_COMPLETE,INS_RTKFIXED,37.37048957210,126.72450735141,11.3626,22.3000,-0.1833,0.2491,0.0031,-0.413726161,1.254488863,120.030297293,0.4551,0.3027,0.5696,0.1158,0.0939,0.0773,0.1402,0.1450,5.0349,0f000001,0*52de2f77\n\tsystem status\tnormal 2 28.000000 0 0\trobot status\t325.281563\t39.878827\t11.362600\t-0.413726\t1.254489\t-30.030297\t0.300000\t0.009000\n\t\n15:26:37.2\tlog_raw\tgps_raw\t#INSPVAXA,USB3,0,53.0,FINESTEERING,2107,282415.200,02000000,471d,15824;INS_ALIGNMENT_COMPLETE,INS_RTKFIXED,37.37048882282,126.72450867783,11.3669,22.3000,-0.1974,0.2488,-0.0050,-0.369163180,1.275233001,120.010997524,0.4468,0.2975,0.5625,0.1152,0.0938,0.0768,0.1401,0.1449,5.0346,0f000001,0*63e54e05\n\tsystem status\tnormal 2 28.000000 0 0\trobot status\t325.399055\t39.795664\t11.366900\t-0.369163\t1.275233\t-30.010998\t0.301000\t0.009000\n\t\n15:26:37.7\tlog_raw\tgps_raw\t#INSPVAXA,USB3,0,53.0,FINESTEERING,2107,282415.700,02000000,471d,15824;INS_ALIGNMENT_COMPLETE,INS_RTKFIXED,37.37048807554,126.72451000285,11.3689,22.3000,-0.1889,0.2508,0.0038,-0.308402860,1.363313459,120.035668332,0.4468,0.2975,0.5625,0.1152,0.0938,0.0768,0.1401,0.1449,5.0346,0f000001,0*269cbb1b\n\tsystem status\tnormal 2 28.000000 0 0\trobot status\t325.516423\t39.712723\t11.368900\t-0.308403\t1.363313\t-30.035668\t0.300000\t0.000000\n\t\n15:26:38.2\tlog_raw\tgps_raw\t#INSPVAXA,USB3,0,49.5,FINESTEERING,2107,282416.200,02000000,471d,15824;INS_ALIGNMENT_COMPLETE,INS_RTKFIXED,37.37048732666,126.72451132645,11.3727,22.3000,-0.2024,0.2646,0.0068,-0.344354829,1.559210135,120.006452776,0.4418,0.2949,0.5567,0.1151,0.0940,0.0765,0.1400,0.1448,5.0344,0f000001,0*5f55c88e\n\tsystem status\tnormal 2 28.000000 0 0\trobot status\t325.633666\t39.629604\t11.372700\t-0.344355\t1.559210\t-30.006453\t0.307000\t0.002000\n\t\n15:26:38.7\tlog_raw\tgps_raw\t#INSPVAXA,USB3,0,49.5,FINESTEERING,2107,282416.700,02000000,471d,15824;INS_ALIGNMENT_COMPLETE,INS_RTKFIXED,37.37048655948,126.72451266499,11.3766,22.3000,-0.1941,0.2563,0.0061,-0.377791585,1.578777969,120.002147142,0.4418,0.2949,0.5567,0.1151,0.0940,0.0765,0.1400,0.1448,5.0344,0f000001,0*34897afe\n\tsystem status\tnormal 2 28.000000 0 0\trobot status\t325.752231\t39.544455\t11.376600\t-0.377792\t1.578778\t-30.002147\t0.303000\t0.007000\n\t\n15:26:39.2\tlog_raw\tgps_raw\t\tsystem status\tnormal 2 28.000000 0 0\trobot status\t325.855280\t39.469306\t11.380500\t-0.290945\t1.667739\t-29.924480\t0.258000\t0.066000\n\t\n15:26:39.7\tlog_raw\tgps_raw\t#INSPVAXA,USB3,0,52.5,FINESTEERING,2107,282417.700,02000000,471d,15824;INS_ALIGNMENT_COMPLETE,INS_RTKFIXED,37.37048504382,126.72451529790,11.3842,22.3000,-0.1953,0.2454,0.0181,-0.246271614,1.533033405,119.744385532,0.4392,0.2938,0.5521,0.1151,0.0941,0.0764,0.1399,0.1448,5.0342,0f000001,0*775a7cde\n\tsystem status\tnormal 2 28.000000 0 0\trobot status\t325.985450\t39.376231\t11.384200\t-0.246272\t1.533033\t-29.744386\t0.376000\t-0.093000\n\t\n15:26:40.2\tlog_raw\tgps_raw\t#INSPVAXA,USB3,0,49.5,FINESTEERING,2107,282418.200,02000000,471d,15824;INS_ALIGNMENT_COMPLETE,INS_RTKFIXED,37.37048430161,126.72451659682,11.3895,22.3000,-0.1860,0.2574,0.0118,-0.194523398,1.357517182,119.541638486,0.4391,0.2937,0.5490,0.1153,0.0938,0.0764,0.1398,0.1447,5.0342,0f000001,0*fd6a5a6b\n\tsystem status\tnormal 2 28.000000 0 0\trobot status\t326.100506\t39.293852\t11.389500\t-0.194523\t1.357517\t-29.541638\t0.297000\t0.020000\n\t\n15:26:40.7\tlog_raw\tgps_raw\t#INSPVAXA,USB3,0,49.5,FINESTEERING,2107,282418.700,02000000,471d,15824;INS_ALIGNMENT_COMPLETE,INS_RTKFIXED,37.37048357095,126.72451792235,11.3949,22.3000,-0.1880,0.2631,0.0129,-0.293493198,1.431848983,119.317686848,0.4391,0.2937,0.5490,0.1153,0.0938,0.0764,0.1398,0.1447,5.0342,0f000001,0*f85c4eed\n\tsystem status\tnormal 2 28.000000 0 0\trobot status\t326.217920\t39.212756\t11.394900\t-0.293493\t1.431849\t-29.317687\t0.356000\t-0.054000\n\t\n15:26:41.2\tlog_raw\tgps_raw\t#INSPVAXA,USB3,0,51.5,FINESTEERING,2107,282419.200,02000000,471d,15824;INS_ALIGNMENT_COMPLETE,INS_RTKFIXED,37.37048282849,126.72451926994,11.3994,22.3000,-0.1790,0.2403,0.0146,-0.323412826,1.420573693,119.067840661,0.4387,0.2935,0.5464,0.1153,0.0936,0.0764,0.1397,0.1447,5.0349,0f000001,0*dfe7d2ed\n\tsystem status\tnormal 2 28.000000 0 0\trobot status\t326.337287\t39.130349\t11.399400\t-0.323413\t1.420574\t-29.067841\t0.253000\t0.069000\n\t\n15:26:41.7\tlog_raw\tgps_raw\t#INSPVAXA,USB3,0,51.5,FINESTEERING,2107,282419.700,02000000,471d,15824;INS_ALIGNMENT_COMPLETE,INS_RTKFIXED,37.37048208962,126.72452059781,11.4036,22.3000,-0.1738,0.2412,0.0141,-0.294957453,1.425673265,118.815782482,0.4387,0.2935,0.5464,0.1153,0.0936,0.0764,0.1397,0.1447,5.0349,0f000001,0*b9942f72\n\tsystem status\tnormal 2 27.900000 0 0\trobot status\t326.454908\t39.048342\t11.403600\t-0.294957\t1.425673\t-28.815782\t0.311000\t-0.012000\n\t\n15:26:42.2\tlog_raw\tgps_raw\t#INSPVAXA,USB3,0,50.5,FINESTEERING,2107,282420.200,02000000,471d,15824;INS_ALIGNMENT_COMPLETE,INS_RTKFIXED,37.37048136193,126.72452192165,11.4068,22.3000,-0.1787,0.2514,0.0118,-0.301136981,1.598998965,118.572497576,0.4423,0.2941,0.5460,0.1156,0.0933,0.0766,0.1396,0.1447,5.0359,0f000001,0*0dbcadaf\n\tsystem status\tnormal 2 28.000000 0 0\trobot status\t326.572171\t38.967575\t11.406800\t-0.301137\t1.598999\t-28.572498\t0.268000\t0.053000\n\t\n15:26:42.7\tlog_raw\tgps_raw\t#INSPVAXA,USB3,0,50.5,FINESTEERING,2107,282420.700,02000000,471d,15824;INS_ALIGNMENT_COMPLETE,INS_RTKFIXED,37.37048063557,126.72452326406,11.4104,22.3000,-0.1682,0.2469,0.0144,-0.349485700,1.489707131,118.312804770,0.4423,0.2941,0.5460,0.1156,0.0933,0.0766,0.1396,0.1447,5.0359,0f000001,0*9bf849d5\n\tsystem status\tnormal 2 27.900000 0 0\trobot status\t326.691080\t38.886955\t11.410400\t-0.349486\t1.489707\t-28.312805\t0.332000\t-0.042000\n\t\n15:26:43.2\tlog_raw\tgps_raw\t#INSPVAXA,USB3,0,48.0,FINESTEERING,2107,282421.200,02000000,471d,15824;INS_ALIGNMENT_COMPLETE,INS_RTKFIXED,37.37047991282,126.72452459987,11.4134,22.3000,-0.1640,0.2507,0.0070,-0.436089069,1.502424265,118.039794860,0.4455,0.2944,0.5457,0.1157,0.0930,0.0767,0.1395,0.1446,5.0372,0f000001,0*71ca6260\n\tsystem status\tnormal 2 27.900000 0 0\trobot status\t326.809404\t38.806737\t11.413400\t-0.436089\t1.502424\t-28.039795\t0.205000\t0.144000\n\t\n15:26:43.7\tlog_raw\tgps_raw\t#INSPVAXA,USB3,0,48.0,FINESTEERING,2107,282421.700,02000000,471d,15824;INS_ALIGNMENT_COMPLETE,INS_RTKFIXED,37.37047920210,126.72452588480,11.4143,22.3000,-0.1661,0.2579,0.0075,-0.445939557,1.526205768,117.767448761,0.4455,0.2944,0.5457,0.1157,0.0930,0.0767,0.1395,0.1446,5.0372,0f000001,0*bff7dfe5\n\tsystem status\tnormal 2 27.900000 0 0\trobot status\t326.923221\t38.727853\t11.414300\t-0.445940\t1.526206\t-27.767449\t0.346000\t-0.045000\n\t\n15:26:44.2\tlog_raw\tgps_raw\t#INSPVAXA,USB3,0,52.0,FINESTEERING,2107,282422.200,02000000,471d,15824;INS_ALIGNMENT_COMPLETE,INS_RTKFIXED,37.37047849051,126.72452721632,11.4160,22.3000,-0.1641,0.2604,0.0088,-0.542046801,1.417066343,117.580039835,0.4474,0.2945,0.5457,0.1156,
